vi "my_gpib_write.vi"(0 "address string":string, 5 "data":string, 11 "error in":errorcluster) -> (15 "error out":errorcluster)   [LabVIEW 2019]
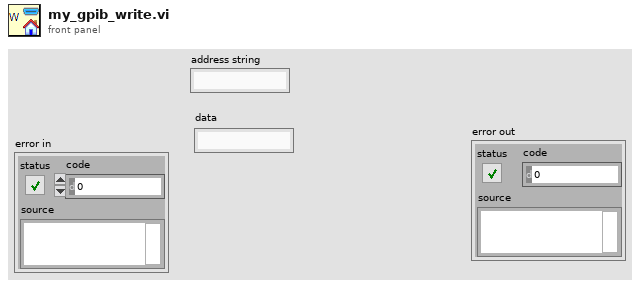
[diagram p1: front panel]
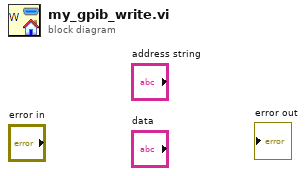
[diagram p0: block diagram]
diagram:
